vi "Dialog Window Setup.vi"(7 "Action":enum16{"Pre-Populate", "Post-Populate"}(ring), 8 "error in":errorcluster, 10 "Dialog VI Ref In [Parent]":refnum<vi>, 11 "Align-to Window Ref":refnum<vi>) -> (0 "error out":errorcluster, 2 "Dialog VI Ref Out":refnum<vi>)   [LabVIEW 2023]
doc: "Pre-populate mode opens the FP in a hidden state, aligns the window to the calling VI (if ref wired in), sets pane origina of all panes, and sets the behavior of the reightmost splitter, which divides the viewed area of the FP from the developer's area.\n\nAfter running prepopulate, you can continue to set up other FP features before running this VI in post-poluate mode, which maes the FP visible and active. \n\nAlign Dialog to a scripted block diagram window, prepare dialog FP (resizing) and open it for view. If Dialog ref is not passesd in it's assumed to be the parent of this VI."
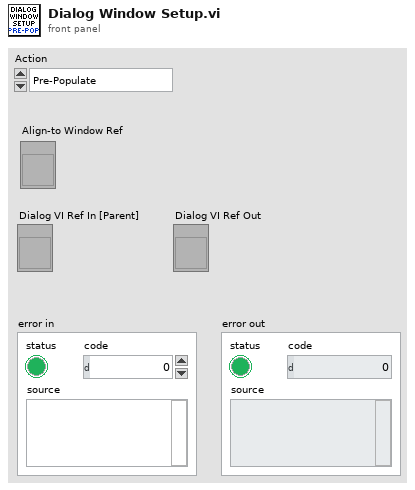
[diagram p1: front panel]
types:
  T1 = enum32{"Invalid", "Standard", "Closed", "Hidden", "Minimized", "Maximized"}
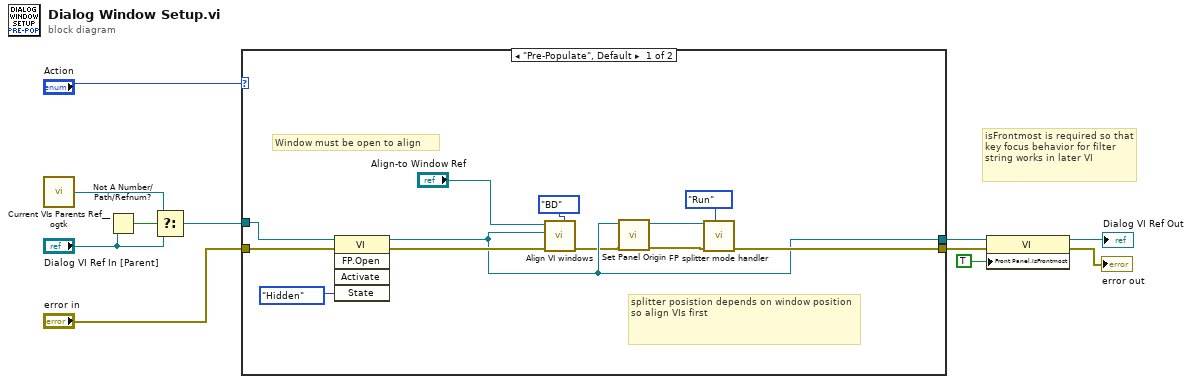
[diagram p0: block diagram]
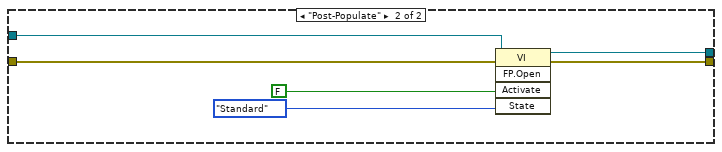
[diagram p2: hidden frame]
diagram:
  # "isFrontmost is required so that key focus behavior for filter string works in later VI"
  n1 = call <userlib>:"Current VIs Parents Ref__ogtk.vi"() -> ("Calling VI's Reference"=w10:refnum<vi>)  [unwired: 2 in]
  n2 = Not A Number/Path/Refnum?(number/path/refnum="Dialog VI Ref In [Parent]") -> (NaN/Path/Refnum?=w7:bool)
  n3 = Select(t=w10, s=w7, f="Dialog VI Ref In [Parent]") -> (s? t:f=w9:refnum<vi>)
  n4 = case shown="\"Pre-Populate\", Default" "Action" {
    tunnel: [w15 w27] -> w3
    tunnel: [w19 w29] -> w5
    tunnel: w9 -> [w22 w24]
    tunnel: "error in" -> [w21 w25]
    frame "Pre-Populate", Default {
      # "splitter posistion depends on window position so align VIs first"
      # "Window must be open to align"
      n5 = invoke class="VI" method="FP.Open"(reference=w22, error in=w21, "State"=T1."Hidden") -> (reference out=w15:refnum<vi>, error out=w18:errorcluster)  [unwired: 2 in, 3 out]
      n6 = call "Align VI windows.vi"("Align to"=enum16{"FP", "BD"}."BD", "error in"=w18, "VI to Move Ref"=w15, "Stationary VI Ref"="Align-to Window Ref") -> ("error out"=w14:errorcluster)  [unwired: 7 in]
      n7 = call "Set Panel Origin.vi"("error in"=w14, "VI Ref In"=w15) -> ("error out"=w12:errorcluster, "VI Ref Out"=w13:refnum<vi>)  [unwired: 8 in]
      n8 = call "FP splitter mode handler.vi"("Mode"=enum16{"Run", "Development"}."Run", "error in"=w12, "VI Ref In"=w13) -> ("error out"=w19:errorcluster)  [unwired: 7 in, 1 out]
    }
    frame "Post-Populate" {
      n9 = invoke class="VI" method="FP.Open"(reference=w24, error in=w25, "Activate"=FALSE ("Activate?"), "State"=T1."Standard") -> (reference out=w27:refnum<vi>, error out=w29:errorcluster)  [unwired: 1 in, 3 out]
    }
  }
  n10 = property class="VI"(reference=w3, error in=w5, "Front Panel.IsFrontmost"=TRUE ("Front Panel Window:Is Frontmost")) -> (reference out=→"Dialog VI Ref Out":refnum<vi>, error out=→"error out":errorcluster)
